vi "EjercicioOndas.vi"() -> ()   [LabVIEW 2020]
uses:
  <vilib>/measure/NI_MABase.lvlib
panel:
  out "Waveform Graph":waveform(dbl)[](graph)
  in  "stop":bool
  in  "Frecuencia f1":dbl(knob) scale=0.0..10.0
  in  "Amplitud f1":dbl(knob) scale=0.0..10.0
  in  "Fase f1":dbl(knob) scale=-100.0..100.0
  in  "Frecuencia f3":dbl(knob) scale=0.0..10.0
  in  "Frecuencia f2":dbl(knob) scale=0.0..10.0
  in  "Amplitud f2":dbl(knob) scale=0.0..10.0
  in  "Fase f2":dbl(knob) scale=-100.0..100.0
  in  "Fase f3":dbl(knob) scale=-100.0..100.0
  in  "Amplitud f3":dbl(knob) scale=0.0..10.0
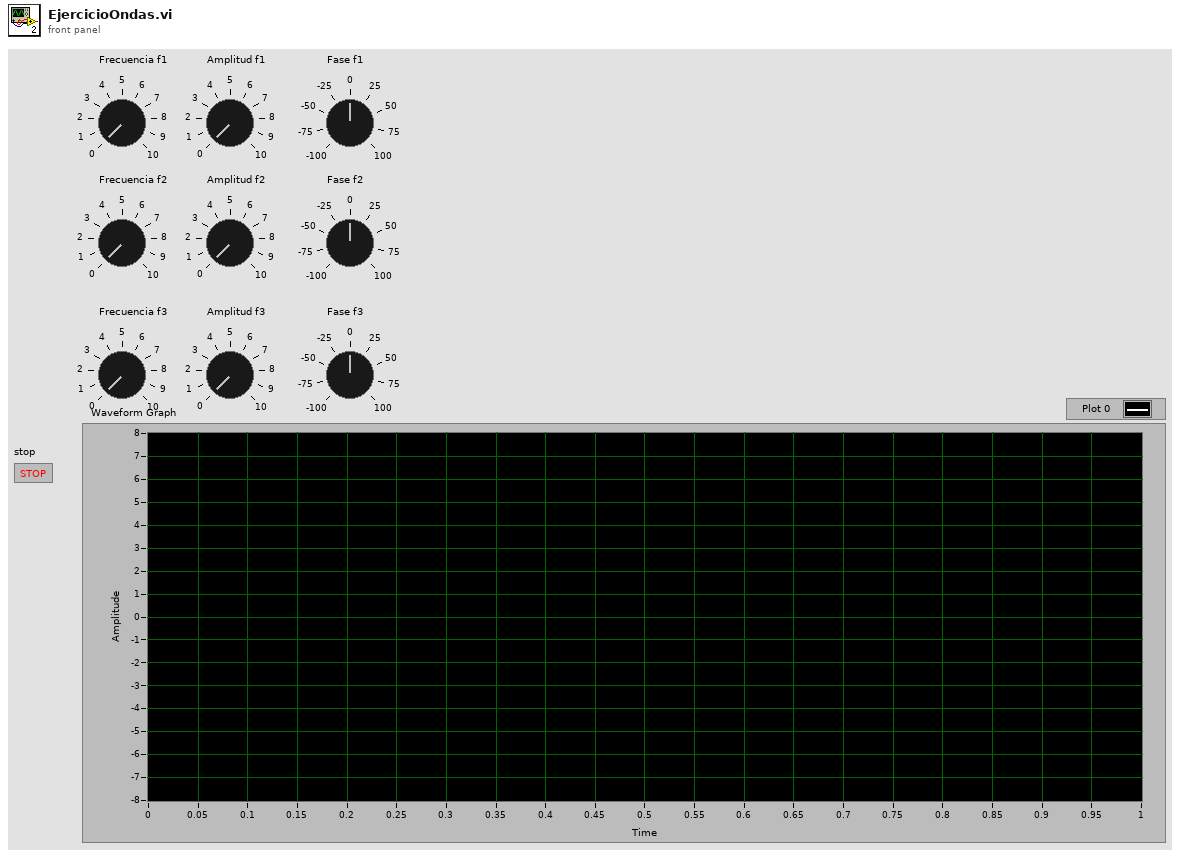
[diagram p1: front panel]
types:
  T1 = enum16{"Sine Wave", "Triangle Wave", "Square Wave"}
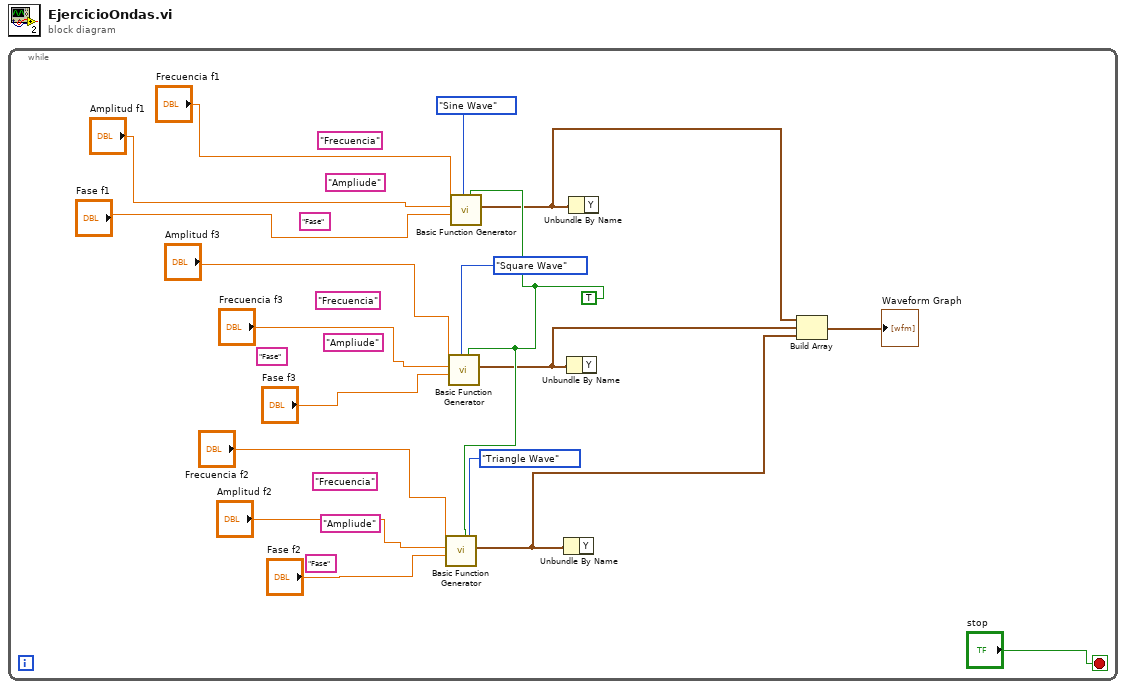
[diagram p0: block diagram]
diagram:
  n1 = while {
    stop <- "stop" stop-if-true
    w6 = TRUE
    (unwired) "Fase"
    (unwired) "Ampliude"
    (unwired) "Frecuencia"
    (unwired) "Fase"
    (unwired) "Ampliude"
    (unwired) "Frecuencia"
    (unwired) "Fase"
    (unwired) "Ampliude"
    (unwired) "Frecuencia"
    n2 = call <vilib>:"Basic Function Generator.vi"("reset signal"=w6, "signal type"=enum16{"Sine Wave", "Triangle Wave"}."Triangle Wave", "phase"="Fase f2", "amplitude"="Amplitud f2", "frequency"="Frecuencia f2") -> ("signal out"=w1:waveform(dbl))  [unwired: 4 in, 2 out]
    n3 = call <vilib>:"Basic Function Generator.vi"("reset signal"=w6, "signal type"=T1."Square Wave", "phase"="Fase f3", "amplitude"="Frecuencia f3", "frequency"="Amplitud f3") -> ("signal out"=w3:waveform(dbl))  [unwired: 4 in, 2 out]
    n4 = call <vilib>:"Basic Function Generator.vi"("reset signal"=w6, "signal type"=enum16{"Sine Wave"}."Sine Wave", "phase"="Fase f1", "amplitude"="Amplitud f1", "frequency"="Frecuencia f1") -> ("signal out"=w4:waveform(dbl))  [unwired: 4 in, 2 out]
    n5 = Unbundle By Name(w1) -> ()  [unwired: 1 out]
    n6 = Unbundle By Name(w3) -> ()  [unwired: 1 out]
    n7 = Unbundle By Name(w4) -> ()  [unwired: 1 out]
    n8 = Build Array(w4, w3, w1) -> (→"Waveform Graph":waveform(dbl)[])
  }
